vi "lab2.vi"() -> ()   [LabVIEW 2020]
panel:
  out "Measured Current":sgl
  out "Measured Voltage":sgl
  in  "Output Current":dbl=1.0
  in  "Output State":u16(ring) items=["OFF", "ON"]
  in  "Channel Control":u16(ring)=1 items=["N/A", "Channel 1", "Channel 2", "Channel 3"]
  out "VISA resource name out":refnum<visa-resource-name>
  in  "Reset? (T: Yes)":bool=TRUE
  in  "VISA resource name":refnum<visa-resource-name>
  in  "min(V) 2":dbl
  in  "max(V) 2":dbl
  in  "step(V) 2":dbl
  out "V":dbl[](array[numeric])
  out "I":dbl[](array[numeric])
  out "XY Graph":cluster{"I":dbl[], "V":dbl[]}(graph)
  out "Measurements":dbl
  in  "Auto Zero (0: Enable)":u32(ring) items=["Enable", "Disable", "Once"]
  in  "Auto Range (T: Enable)":bool=TRUE
  in  "Function (0: Voltage DC)":i32(ring) items=[" Voltage DC", "Voltage AC", "Current DC", "Current AC", "Resistance", "4-wire Resistance", "Diode", "Capacitance", "Temperature", "Continuity", "Frequency", "Period", "Voltage Ratio", "Digitize Voltage", "Digitize Current"]
  in  "Manual Range (0)":dbl
  in  "VISA resource name 2":refnum<visa-resource-name>
  # "电压源 2231A-30-A"
  # "万用表 DMM6500"
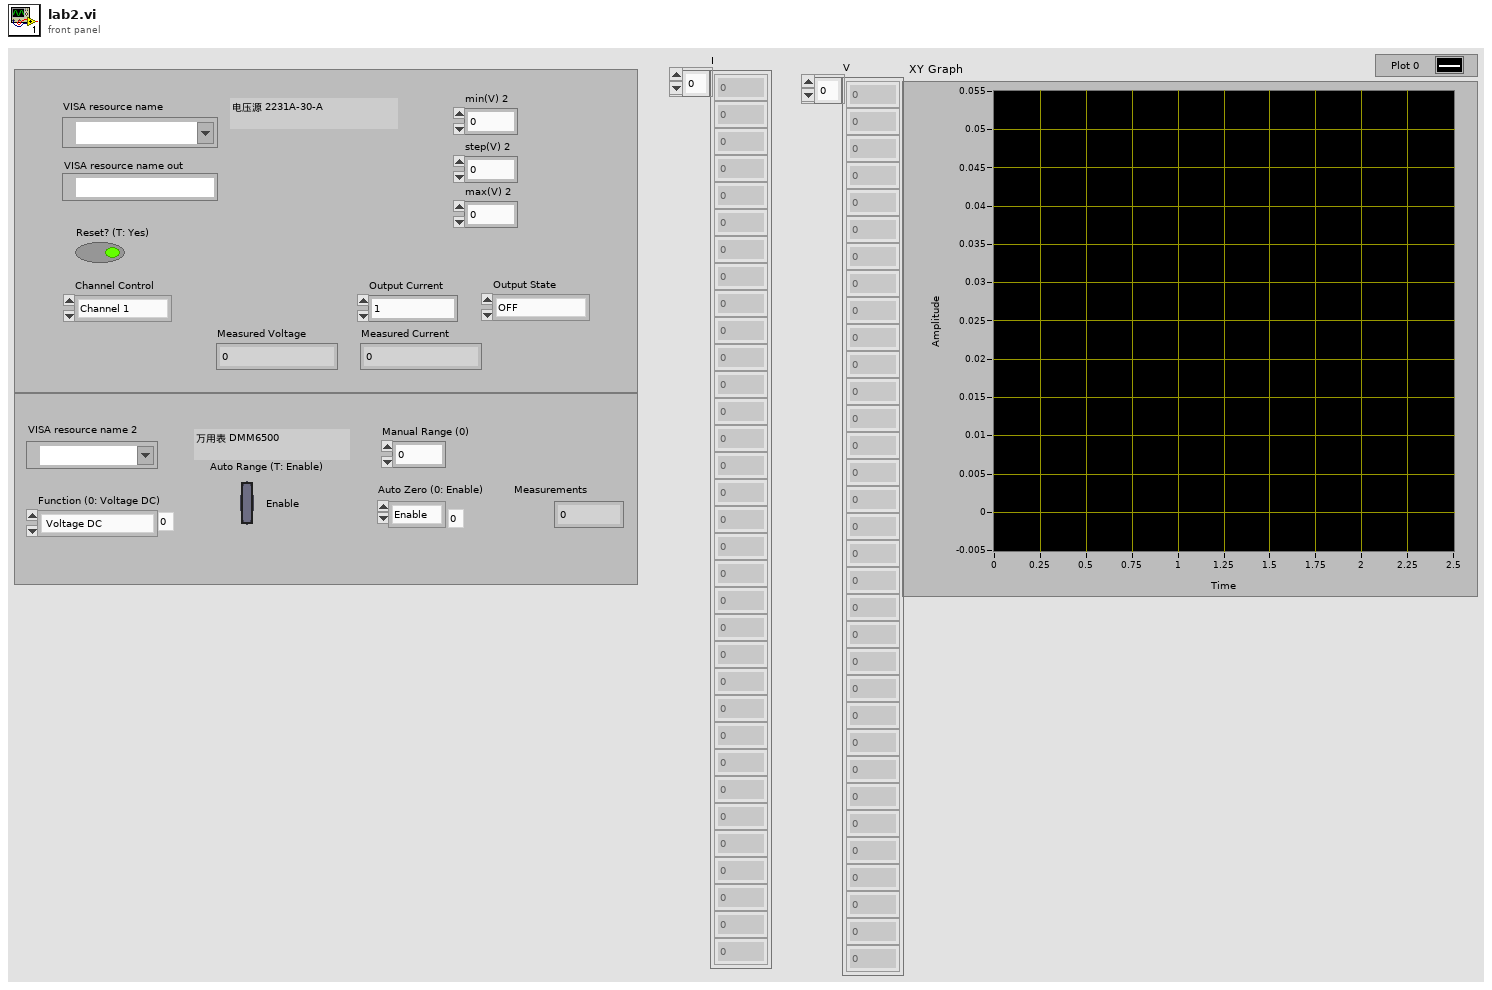
[diagram p1: front panel]
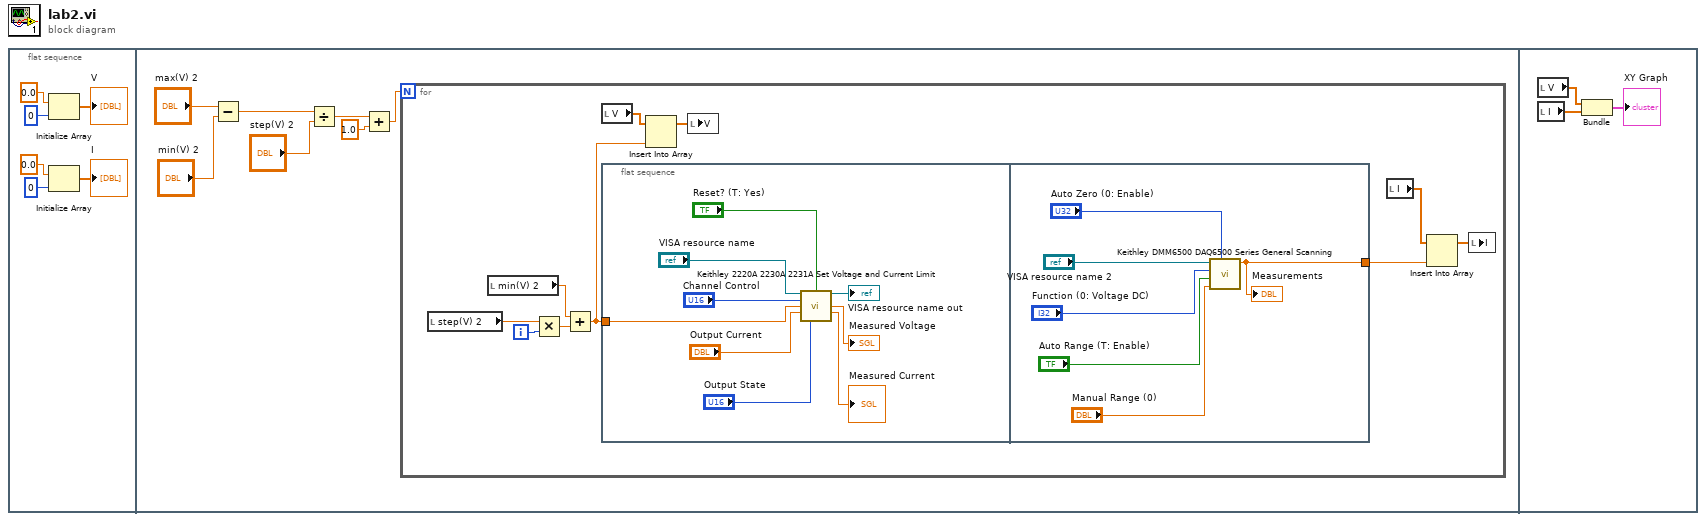
[diagram p0: block diagram]
diagram:
  n1 = flat-sequence {
    frame #0 {
      n2 = Initialize Array(0.0 ("element"), 0 ("dimension size")) -> (→"V":dbl[])
      n3 = Initialize Array(0.0 ("element"), 0 ("dimension size")) -> (→"I":dbl[])
    }
    frame #1 {
      n4 = Subtract(x="max(V) 2", y="min(V) 2") -> (x-y=w11:dbl)
      n5 = Divide(x=w11, y="step(V) 2") -> (x/y=w9:dbl)
      n6 = Add(x=w9, y=1.0) -> (x+y=w7:dbl)
      n7 = for {
        N: w7 -> [_]
        i -> [w21]
        n8 = local read "step(V) 2"() -> (w20:dbl)
        n9 = local read "min(V) 2"() -> (w22:dbl)
        n10 = Multiply(x=w20, y=w21) -> (x*y=w19:dbl)
        n11 = Add(x=w22, y=w19) -> (x+y=w17:dbl)
        n12 = local read "V"() -> (w23:dbl[])
        n13 = flat-sequence {
          tunnel: w17 -> [w24]
          tunnel: [w33] -> w14
          frame #0 {
            n14 = call "Keithley 2220A 2230A 2231A Set Voltage and Current Limit.vi"("VISA resource name"="VISA resource name", "Reset? (T: Yes)"="Reset? (T: Yes)", "Channel Control"="Channel Control", "Supply Voltage"=w24, "Output Current"="Output Current", "Output State"="Output State") -> ("VISA resource name out"=→"VISA resource name out":refnum<visa-resource-name>, "Measured Voltage"=→"Measured Voltage":sgl, "Measured Current"=→"Measured Current":sgl)  [unwired: 6 in, 1 out]
          }
          frame #1 {
            n15 = call "Keithley DMM6500 DAQ6500 Series General Scanning.vi"("Auto Zero (0: Enable)"="Auto Zero (0: Enable)", "Manual Range (0)"="Manual Range (0)", "Auto Range (T: Enable)"="Auto Range (T: Enable)", "Function (0: Voltage DC)"="Function (0: Voltage DC)", "VISA resource name"="VISA resource name 2") -> ("Measurements"=w33:dbl)  [unwired: 6 in]
            "Measurements" <- w33
          }
        }
        n16 = Insert Into Array(array=w23, new element=w17) -> (w18:dbl[])  [unwired: 1 in]
        n17 = local write "V"(w18) -> ()
        n18 = local read "I"() -> (w16:dbl[])
        n19 = Insert Into Array(array=w16, new element=w14) -> (w15:dbl[])  [unwired: 1 in]
        n20 = local write "I"(w15) -> ()
      }
    }
    frame #2 {
      n21 = local read "V"() -> (w40:dbl[])
      n22 = local read "I"() -> (w39:dbl[])
      n23 = Bundle("V"=w40, "I"=w39) -> (→"XY Graph":cluster{"V":dbl[], "I":dbl[]})  [unwired: 1 in]
    }
  }
